vi "Bang Bang.vi"() -> ()   [LabVIEW 2020]
panel:
  out "Output":dbl
  in  "Range":dbl
  in  "Setpoint":dbl
  in  "Actual":dbl
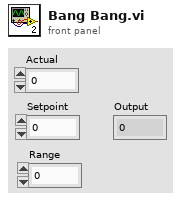
[diagram p1: front panel]
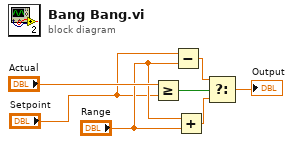
[diagram p0: block diagram]
diagram:
  n1 = Greater Or Equal?(x="Actual", y="Setpoint") -> (x >= y?=w7:bool)
  n2 = Subtract(x="Setpoint", y="Range") -> (x-y=w6:dbl)
  n3 = Add(x="Range", y="Range") -> (x+y=w5:dbl)
  n4 = Select(t=w6, s=w7, f=w5) -> (s? t:f=→"Output":dbl)
